vi "Construct sqlite configuration database queries.vi"(4 "value column":string="value", 6 "name column":string="name", 8 "error in (no error)":errorcluster, 10 "table name":string="configuration", 11 "database path":path) -> (0 "error out":errorcluster, 3 "sqlite-configdb-queries out":refnum<class "sqlite-queries.lvclass">)   [LabVIEW 2020, in "sqlite-queries.lvlib" / "sqlite-queries.lvclass"]
uses:
  sqlite-queries.lvclass
  sqlite-queries.lvclass/sqlite-queries.ctl
  externals/database-interface/IDatabase/IDatabase.lvlib
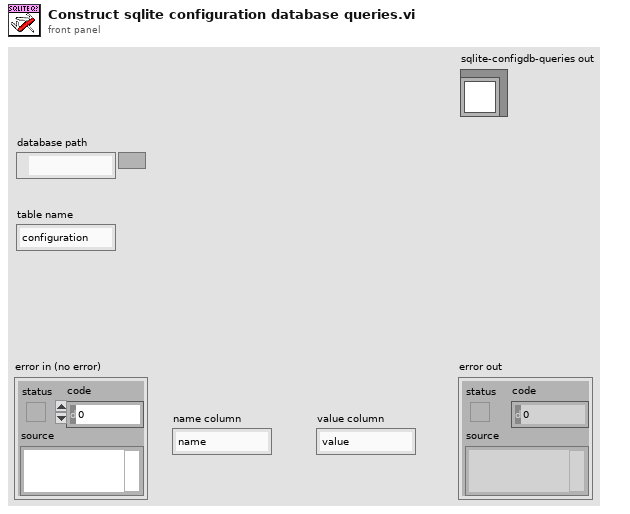
[diagram p1: front panel]
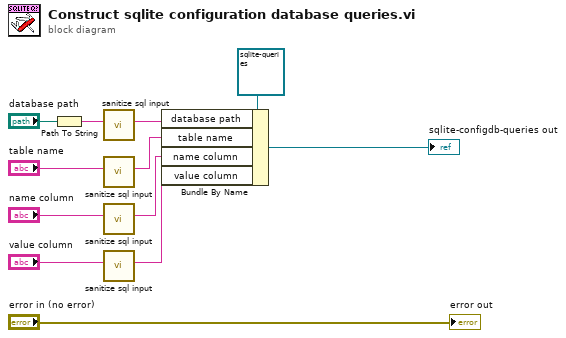
[diagram p0: block diagram]
diagram:
  n1 = Path To String(path="database path") -> (string=w1:string)
  n2 = call "sanitize sql input.vi"("Sting in"=w1) -> ("String out"=w5:string)  [unwired: 8 in, 2 out]
  n3 = call "sanitize sql input.vi"("Sting in"="table name") -> ("String out"=w4:string)  [unwired: 8 in, 2 out]
  n4 = call "sanitize sql input.vi"("Sting in"="name column") -> ("String out"=w3:string)  [unwired: 8 in, 2 out]
  n5 = call "sanitize sql input.vi"("Sting in"="value column") -> ("String out"=w2:string)  [unwired: 8 in, 2 out]
  n6 = Bundle By Name(cluster=refnum<class "sqlite-queries.lvclass"> refnum ("sqlite-configdb-queries in"), "database path"=w5, "table name"=w4, "name column"=w3, "value column"=w2) -> (→"sqlite-configdb-queries out":refnum<class "sqlite-queries.lvclass">)
  "error out" <- "error in (no error)"
